vi "Main.vi"() -> ()   [LabVIEW 2020, in "MeasurementService_Template.lvlib" / "MeasurementService_Template.lvclass"]
uses:
  MeasurementService_Template.lvclass
  typeDefs/Server State Data.ctl
  MeasurementService_Template.lvclass/MeasurementService_Template.ctl
  <vilib>/gRPC/Discovery Client/Discovery_client Class/Discovery_client.lvclass
panel:
  out "Listening Port":i32
  in  "Stop":bool
  in  "Enable Async Mode":bool
  in  "Server Address":string="localhost:50051"
  in  "Server Certificate File (.crt)":path
  in  "Server Key File (.key)":path
  # "Note: If you want the service to auto find the listening port, then enter the port number in \"Server Address\" as 0. Ex: localhost:0"
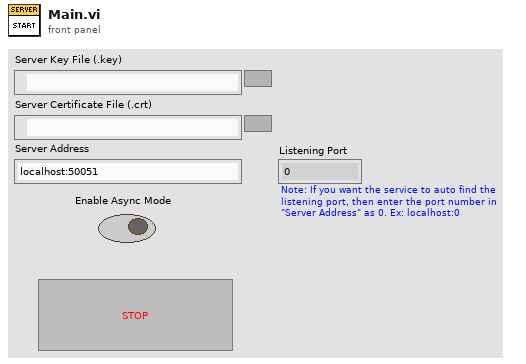
[diagram p1: front panel]
types:
  T1 = typedef "MeasurementService_Template.lvlib/MeasurementService_Template.lvclass/Server State Data.ctl" = cluster{"Data":string}
  T2 = typedef "Discovery_client-release.lvlib/Discovery_client.lvclass/NIMeasurementServices_RegisterServiceResponse_Data.ctl" = cluster{"regisration_id":string}
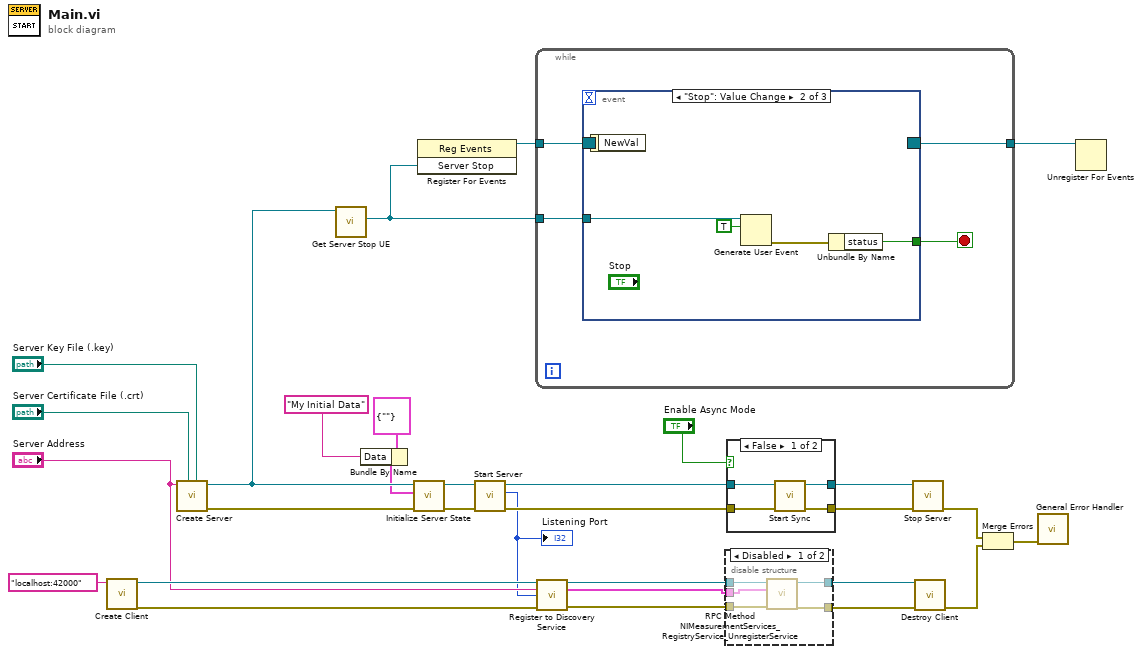
[diagram p0: block diagram]
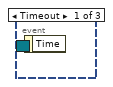
[diagram p3: hidden frame]
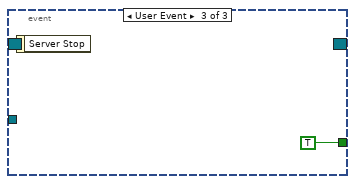
[diagram p4: hidden frame]
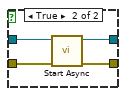
[diagram p5: hidden frame]
diagram:
  n1 = call <vilib>:"Create Client.vi"("address"="localhost:42000") -> ("error out"=w9:errorcluster, "gRPC Client out"=w12:refnum<class "Discovery_client.lvclass">)  [unwired: 9 in]
  n2 = call "Create Server.vi"("Server Key File (.key)"="Server Key File (.key)", "Server Certificate File (.crt)"="Server Certificate File (.crt)", "Server Address"="Server Address") -> ("error out"=w20:errorcluster, "gRPC Server out"=w17:refnum<class "MeasurementService_Template.lvclass">)  [unwired: 7 in]
  n3 = call "Get Server Stop UE.vi"("OOP Server in"=w17) -> ("Server Stop"=w21:refnum<user-event>)  [unwired: 9 in, 1 out]
  n4 = Bundle By Name(cluster=T1 {"Data"=""} ("Initial State"), "Data"="My Initial Data") -> (w15:T1)
  n5 = call "Initialize Server State.vi"("error in (no error)"=w20, "Initial State"=w15, "gRPC Server in"=w17) -> ("error out"=w19:errorcluster, "gRPC Server out"=w18:refnum<class "MeasurementService_Template.lvclass">)  [unwired: 7 in]
  n6 = register-events(w21) -> (reference out=w23:refnum<event-registration>)  [unwired: 2 in, 1 out]
  n7 = call "Start Server.vi"("error in (no error)"=w19, "gRPC Server in"=w18) -> ("error out"=w30:errorcluster, "Listening Port"=w10:i32, "gRPC Server out"=w29:refnum<class "MeasurementService_Template.lvclass">)  [unwired: 7 in]
  "Listening Port" <- w10
  n8 = while {
    tunnel: w21 -> [w34]
    tunnel: w23 -> [w33]
    tunnel: [w31] -> w22
    stop <- w32 stop-if-true
    n9 = event shown="[1] \"Stop\": Value Change" {
      selector: w33 -> [_ _ _]
      dyn-events: [_ _ _] -> w31
      timeout: _ -> [_ _ _]
      tunnel: w34 -> [_ w38 _]
      tunnel: [_ w35 TRUE] -> w32
      event Timeout {
        n10 = event-data() -> ()  [unwired: 1 in, 1 out]
      }
      event "Stop": Value Change {
        n11 = event-data() -> ()  [unwired: 1 in, 1 out]
        n12 = Generate User Event(user event=w38, event data cluster=TRUE ("event data")) -> (error out=w36:errorcluster)  [unwired: 2 in, 1 out]
        n13 = Unbundle By Name(w36) -> ("status"=w35:bool)
      }
      event User Event {
        n14 = event-data() -> ()  [unwired: 1 in, 1 out]
      }
    }
  }
  n15 = call "Register to Discovery Service.vi"("gRPC Client in"=w12, "Server Address"="Server Address", "Listening Port"=w10, "error in (no error)"=w9) -> ("gRPC Client"=w8:refnum<class "Discovery_client.lvclass">, "Response Data"=w4:T2, "error out"=w5:errorcluster)  [unwired: 9 in]
  n16 = disable-structure shown="Disabled" {
    disable-tunnel: w8 -> [w44 w46]
    disable-tunnel: [w43 w46] -> w7
    disable-tunnel: [w42 w45] -> w6
    disable-tunnel: w5 -> [w41 w45]
    disable-tunnel: w4 -> [w40 _]
    frame Disabled {
      n17 = call <vilib>:"RPC Method NIMeasurementServices_RegistryService_UnregisterService.vi"("error in (no error)"=w41, "Request Data"=w40, "gRPC Client in"=w44) -> ("error out"=w42:errorcluster, "gRPC Client out"=w43:refnum<class "Discovery_client.lvclass">)  [unwired: 6 in, 1 out]
    }
    frame Enabled {
    }
  }
  n18 = case shown="False" "Enable Async Mode" {
    tunnel: w30 -> [w50 w54]
    tunnel: w29 -> [w49 w53]
    tunnel: [w48 w51] -> w28
    tunnel: [w47 w52] -> w27
    frame False {
      n19 = call "Start Sync.vi"("error in (no error)"=w50, "gRPC Server in"=w49) -> ("error out"=w48:errorcluster, "gRPC Server out"=w47:refnum<class "MeasurementService_Template.lvclass">)  [unwired: 8 in]
    }
    frame True {
      n20 = call "Start Async.vi"("error in (no error)"=w54, "gRPC Server in"=w53) -> ("error out"=w51:errorcluster, "gRPC Server out"=w52:refnum<class "MeasurementService_Template.lvclass">)  [unwired: 8 in]
    }
  }
  n21 = call "Stop Server.vi"("error in (no error)"=w28, "gRPC Server in"=w27) -> ("error out"=w3:errorcluster)  [unwired: 9 in]
  n22 = call <vilib>:"Destroy Client.vi"("error in (no error)"=w6, "gRPC Client in"=w7) -> ("error out"=w2:errorcluster)  [unwired: 8 in, 1 out]
  n23 = Merge Errors(w3, w2) -> (w1:errorcluster)
  n24 = call <vilib>:"General Error Handler.vi"("error in (no error)"=w1) -> ()  [unwired: 10 in, 5 out]
  n25 = Unregister For Events(event registration refnum=w22) -> ()  [unwired: 1 in, 1 out]
